vi "Set Source Only.vi"(8 "error in (no error)":errorcluster, 11 "VI in":refnum<vi>) -> (0 "error out":errorcluster, 3 "VI out":refnum<vi>)   [LabVIEW 2019, in "gRPC Template Creation Utility.lvlib"]
uses:
  gRPC Template Creation Utility.lvlib
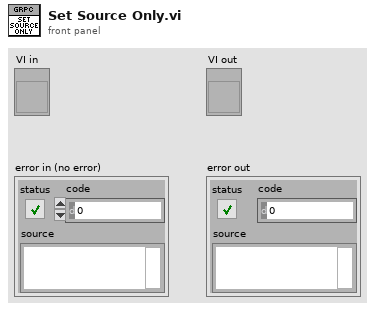
[diagram p1: front panel]
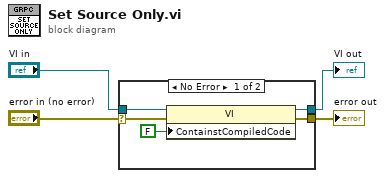
[diagram p0: block diagram]
diagram:
  n1 = case shown="No Error" "error in (no error)" {
    selector: "error in (no error)" -> [w6 w11]
    tunnel: [w8 w11] -> w3
    tunnel: "VI in" -> [w5 w10]
    tunnel: [w9 w10] -> w1
    frame No Error {
      n2 = property class="VI"(reference=w5, error in=w6, "ContainstCompiledCode"=FALSE ("Contains Compiled Code")) -> (reference out=w9:refnum<vi>, error out=w8:errorcluster)
    }
    frame Error {
    }
  }
  "error out" <- w3
  "VI out" <- w1
